vi "DriverControls.vi"(9 "AngleJoystickName":string, 10 "LifterJoystickName":string, 11 "CaseInput":string) -> ()   [LabVIEW 2013]
uses:
  <vilib>/Rock Robotics/WPI/Joystick/WPI_JoystickGetSetRefNum.vi
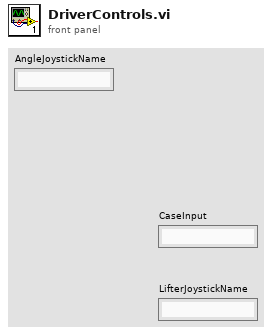
[diagram p1: front panel]
types:
  T1 = typedef "WPI_JoystickDevRef.ctl" = cluster{"Device":T2}
  T2 = typedef "WPI_JoystickDeviceEnum.ctl" = enum16{"USB 1", "USB 2", "USB 3", "USB 4", "Kinect 1", "Kinect 2"}
  T3 = typedef "WPI_JoystickButtonState.ctl" = cluster{"Button 1":bool, "Button 2":bool, "Button 3":bool, "Button 4":bool, "Button 5":bool, "Button 6":bool, "Button 7":bool, "Button 8":bool, "Button 9":bool, "Button 10":bool, "Button 11":bool, "Button 12":bool}
  T4 = typedef "WPI_MotorControlDeviceRef.ctl" = cluster{"DeviceStatus":errorcluster, "Type":enum16{"PWM", "CAN"}, "PWM":cluster{"Digital Module":T5, "PWM Channel":T6, "DeadBand":T7}, "CAN":cluster{"Device Number":u8, "Control Mode":T8, "Semaphore":T9, "Max Vout":dbl}, "Invert":bool, "TransformRef":T10, "InvTransformRef":T10}
  T5 = typedef "FPGA_TypedefDigitalModule.ctl" = enum16{"Digital Module 1", "Digital Module 2"}
  T6 = typedef "FPGA_DIOPWMChannel.ctl" = enum8{"PWM 1", "PWM 2", "PWM 3", "PWM 4", "PWM 5", "PWM 6", "PWM 7", "PWM 8", "PWM 9", "PWM 10", "Invalid"}
  T7 = typedef "WPI_PWMDeadband.ctl" = cluster{"Name":string, "maxPositivePwm":i32, "minPositivePwm":i32, "centerPwm":i32, "maxNegativePwm":i32, "minNegativePwm":i32, "angularRange":u16}
  T8 = typedef "WPI_CANJaguar_ControlMode.ctl" = enum8{"Percent VBus", "Current", "Speed", "Position", "Voltage"}
  T9 = typedef "Semaphore RefNum" = refnum<k1>
  T10 = typedef "WPI_PWMTransform_ConPane.ctl" = refnum<vi>
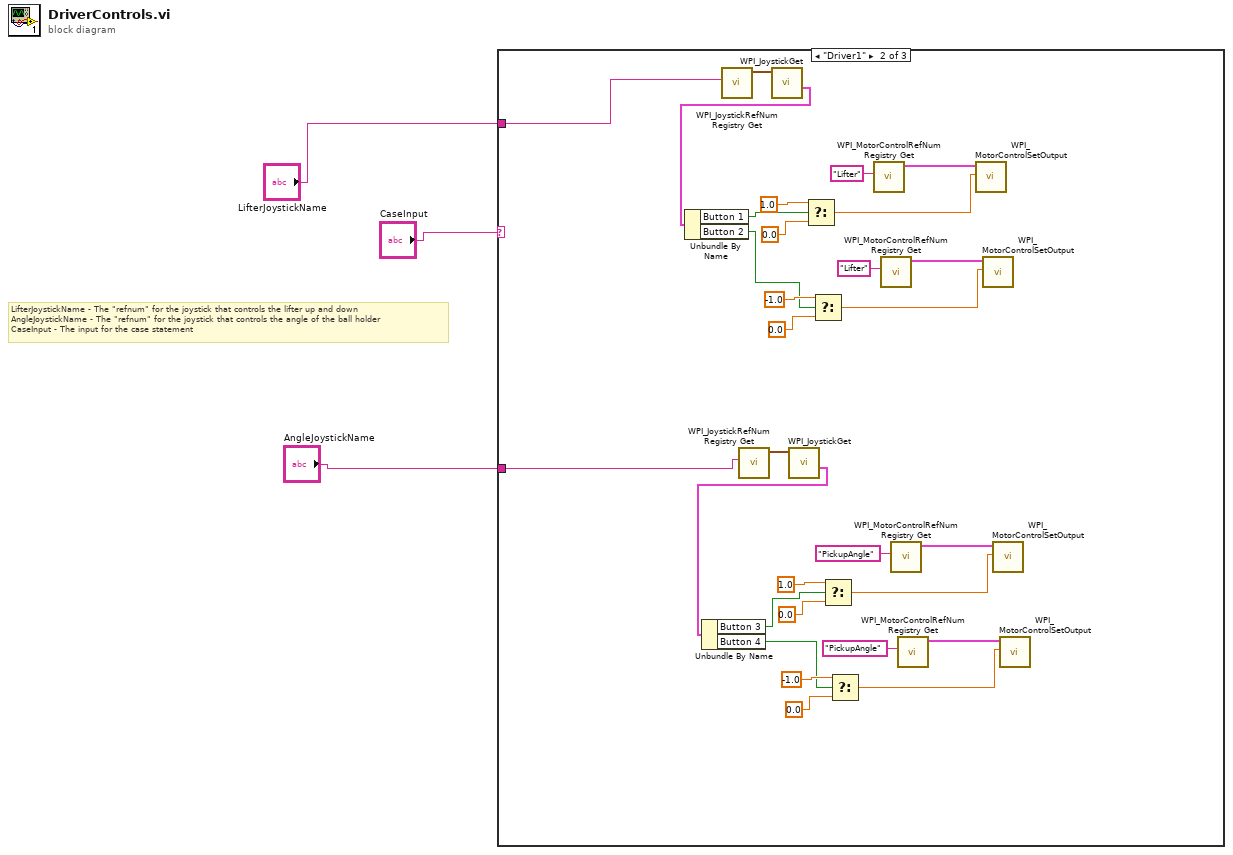
[diagram p0: block diagram]
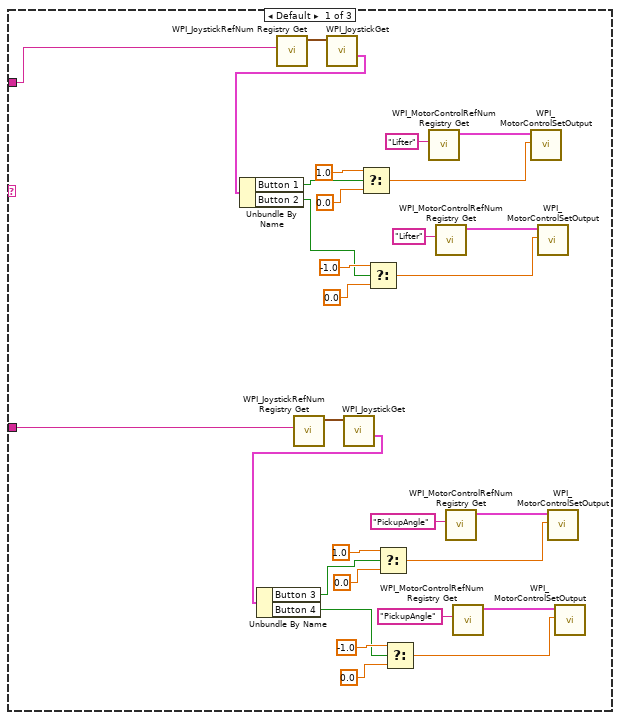
[diagram p2: hidden frame]
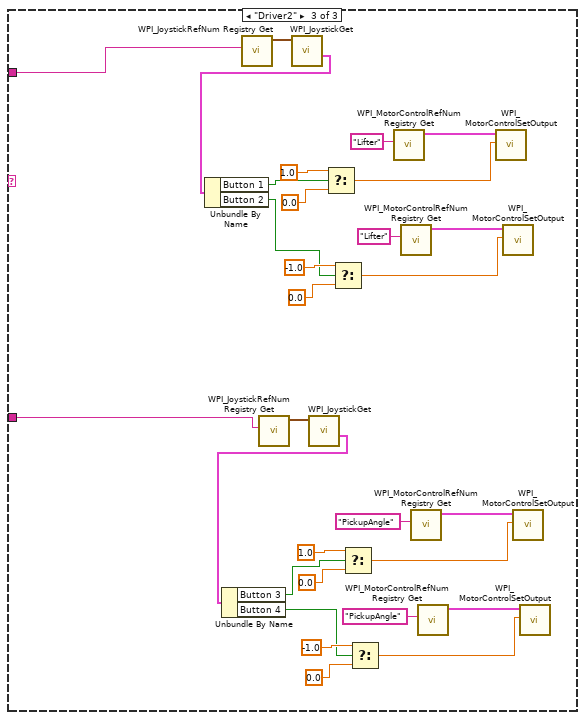
[diagram p3: hidden frame]
diagram:
  # "LifterJoystickName - The \"refnum\" for the joystick that controls the lifter up and down\nAngleJoystickName - The \"refnum\" for the joystick that controls the angle of the ball holder\nCaseInput - The input for the case statement"
  n1 = case shown="\"Driver1\"" "CaseInput" {
    tunnel: "LifterJoystickName" -> [w5 w35 w65]
    tunnel: "AngleJoystickName" -> [w4 w34 w64]
    frame Default {
      n2 = call <vilib>:"WPI_JoystickRefNum Registry Get.vi"("refnum name"=w5) -> ("JoystickDevRef"=w33:T1)  [unwired: 1 in, 9 out]
      n3 = call <vilib>:"WPI_JoystickRefNum Registry Get.vi"("refnum name"=w4) -> ("JoystickDevRef"=w19:T1)  [unwired: 1 in, 9 out]
      n4 = call <vilib>:"WPI_JoystickGet.vi"("JoystickDevRef"=w33) -> ("Buttons"=w32:T3)  [unwired: 1 in, 5 out]
      n5 = Unbundle By Name(w32) -> ("Button 1"=w29:bool, "Button 2"=w20:bool)
      n6 = call <vilib>:"WPI_JoystickGet.vi"("JoystickDevRef"=w19) -> ("Buttons"=w18:T3)  [unwired: 1 in, 5 out]
      n7 = Unbundle By Name(w18) -> ("Button 3"=w7:bool, "Button 4"=w6:bool)
      n8 = Select(t=1.0, s=w29, f=0.0 ("t")) -> (s? t:f=w28:dbl)
      n9 = Select(t=-1.0, s=w20, f=0.0 ("t")) -> (s? t:f=w23:dbl)
      n10 = Select(t=1.0, s=w7, f=0.0 ("t")) -> (s? t:f=w15:dbl)
      n11 = Select(t=-1.0, s=w6, f=0.0 ("t")) -> (s? t:f=w10:dbl)
      n12 = call <vilib>:"WPI_MotorControlRefNum Registry Get.vi"("refnum name"="Lifter") -> ("MotorControlDevRef"=w30:T4)  [unwired: 9 in, 1 out]
      n13 = call <vilib>:"WPI_MotorControlRefNum Registry Get.vi"("refnum name"="Lifter") -> ("MotorControlDevRef"=w22:T4)  [unwired: 9 in, 1 out]
      n14 = call <vilib>:"WPI_MotorControlRefNum Registry Get.vi"("refnum name"="PickupAngle") -> ("MotorControlDevRef"=w16:T4)  [unwired: 9 in, 1 out]
      n15 = call <vilib>:"WPI_MotorControlRefNum Registry Get.vi"("refnum name"="PickupAngle") -> ("MotorControlDevRef"=w9:T4)  [unwired: 9 in, 1 out]
      n16 = call <vilib>:"WPI_MotorControlSetOutput.vi"("Output"=w28, "MotorControlDevRef"=w30) -> ()  [unwired: 7 in, 3 out]
      n17 = call <vilib>:"WPI_MotorControlSetOutput.vi"("Output"=w23, "MotorControlDevRef"=w22) -> ()  [unwired: 7 in, 3 out]
      n18 = call <vilib>:"WPI_MotorControlSetOutput.vi"("Output"=w15, "MotorControlDevRef"=w16) -> ()  [unwired: 7 in, 3 out]
      n19 = call <vilib>:"WPI_MotorControlSetOutput.vi"("Output"=w10, "MotorControlDevRef"=w9) -> ()  [unwired: 7 in, 3 out]
    }
    frame "Driver1" {
      n20 = call <vilib>:"WPI_JoystickRefNum Registry Get.vi"("refnum name"=w35) -> ("JoystickDevRef"=w63:T1)  [unwired: 1 in, 9 out]
      n21 = call <vilib>:"WPI_JoystickRefNum Registry Get.vi"("refnum name"=w34) -> ("JoystickDevRef"=w49:T1)  [unwired: 1 in, 9 out]
      n22 = call <vilib>:"WPI_JoystickGet.vi"("JoystickDevRef"=w63) -> ("Buttons"=w62:T3)  [unwired: 1 in, 5 out]
      n23 = Unbundle By Name(w62) -> ("Button 1"=w59:bool, "Button 2"=w50:bool)
      n24 = call <vilib>:"WPI_JoystickGet.vi"("JoystickDevRef"=w49) -> ("Buttons"=w48:T3)  [unwired: 1 in, 5 out]
      n25 = Unbundle By Name(w48) -> ("Button 3"=w37:bool, "Button 4"=w36:bool)
      n26 = Select(t=1.0, s=w59, f=0.0 ("t")) -> (s? t:f=w58:dbl)
      n27 = Select(t=-1.0, s=w50, f=0.0 ("t")) -> (s? t:f=w53:dbl)
      n28 = Select(t=1.0, s=w37, f=0.0 ("t")) -> (s? t:f=w45:dbl)
      n29 = Select(t=-1.0, s=w36, f=0.0 ("t")) -> (s? t:f=w40:dbl)
      n30 = call <vilib>:"WPI_MotorControlRefNum Registry Get.vi"("refnum name"="Lifter") -> ("MotorControlDevRef"=w60:T4)  [unwired: 9 in, 1 out]
      n31 = call <vilib>:"WPI_MotorControlRefNum Registry Get.vi"("refnum name"="Lifter") -> ("MotorControlDevRef"=w52:T4)  [unwired: 9 in, 1 out]
      n32 = call <vilib>:"WPI_MotorControlRefNum Registry Get.vi"("refnum name"="PickupAngle") -> ("MotorControlDevRef"=w46:T4)  [unwired: 9 in, 1 out]
      n33 = call <vilib>:"WPI_MotorControlRefNum Registry Get.vi"("refnum name"="PickupAngle") -> ("MotorControlDevRef"=w39:T4)  [unwired: 9 in, 1 out]
      n34 = call <vilib>:"WPI_MotorControlSetOutput.vi"("Output"=w58, "MotorControlDevRef"=w60) -> ()  [unwired: 7 in, 3 out]
      n35 = call <vilib>:"WPI_MotorControlSetOutput.vi"("Output"=w53, "MotorControlDevRef"=w52) -> ()  [unwired: 7 in, 3 out]
      n36 = call <vilib>:"WPI_MotorControlSetOutput.vi"("Output"=w45, "MotorControlDevRef"=w46) -> ()  [unwired: 7 in, 3 out]
      n37 = call <vilib>:"WPI_MotorControlSetOutput.vi"("Output"=w40, "MotorControlDevRef"=w39) -> ()  [unwired: 7 in, 3 out]
    }
    frame "Driver2" {
      n38 = call <vilib>:"WPI_JoystickRefNum Registry Get.vi"("refnum name"=w65) -> ("JoystickDevRef"=w93:T1)  [unwired: 1 in, 9 out]
      n39 = call <vilib>:"WPI_JoystickRefNum Registry Get.vi"("refnum name"=w64) -> ("JoystickDevRef"=w79:T1)  [unwired: 1 in, 9 out]
      n40 = call <vilib>:"WPI_JoystickGet.vi"("JoystickDevRef"=w93) -> ("Buttons"=w92:T3)  [unwired: 1 in, 5 out]
      n41 = Unbundle By Name(w92) -> ("Button 1"=w89:bool, "Button 2"=w80:bool)
      n42 = call <vilib>:"WPI_JoystickGet.vi"("JoystickDevRef"=w79) -> ("Buttons"=w78:T3)  [unwired: 1 in, 5 out]
      n43 = Unbundle By Name(w78) -> ("Button 3"=w67:bool, "Button 4"=w66:bool)
      n44 = Select(t=1.0, s=w89, f=0.0 ("t")) -> (s? t:f=w88:dbl)
      n45 = Select(t=-1.0, s=w80, f=0.0 ("t")) -> (s? t:f=w83:dbl)
      n46 = Select(t=1.0, s=w67, f=0.0 ("t")) -> (s? t:f=w75:dbl)
      n47 = Select(t=-1.0, s=w66, f=0.0 ("t")) -> (s? t:f=w70:dbl)
      n48 = call <vilib>:"WPI_MotorControlRefNum Registry Get.vi"("refnum name"="Lifter") -> ("MotorControlDevRef"=w90:T4)  [unwired: 9 in, 1 out]
      n49 = call <vilib>:"WPI_MotorControlRefNum Registry Get.vi"("refnum name"="Lifter") -> ("MotorControlDevRef"=w82:T4)  [unwired: 9 in, 1 out]
      n50 = call <vilib>:"WPI_MotorControlRefNum Registry Get.vi"("refnum name"="PickupAngle") -> ("MotorControlDevRef"=w76:T4)  [unwired: 9 in, 1 out]
      n51 = call <vilib>:"WPI_MotorControlRefNum Registry Get.vi"("refnum name"="PickupAngle") -> ("MotorControlDevRef"=w69:T4)  [unwired: 9 in, 1 out]
      n52 = call <vilib>:"WPI_MotorControlSetOutput.vi"("Output"=w88, "MotorControlDevRef"=w90) -> ()  [unwired: 7 in, 3 out]
      n53 = call <vilib>:"WPI_MotorControlSetOutput.vi"("Output"=w83, "MotorControlDevRef"=w82) -> ()  [unwired: 7 in, 3 out]
      n54 = call <vilib>:"WPI_MotorControlSetOutput.vi"("Output"=w75, "MotorControlDevRef"=w76) -> ()  [unwired: 7 in, 3 out]
      n55 = call <vilib>:"WPI_MotorControlSetOutput.vi"("Output"=w70, "MotorControlDevRef"=w69) -> ()  [unwired: 7 in, 3 out]
    }
  }
